vi "Motor Transfer.vi"() -> ()   [LabVIEW 2017]
panel:
  in  "Transfer Function Paramters":T1(array[cluster])=[{"Positive"={"Slope"=10.938761399489797, "Intercept"=-2.8907221360051634}, "Negative"={"Slope"=10.353560585244502, "Intercept"=2.6844501013936566}}, {"Positive"={"Slope"=10.727962252753825, "Intercept"=-2.8448867369446544}, "Negative"={"Slope"=10.977250586448044, "Intercept"=2.8878306079303058}}]
  # "Left Wheel"
  # "Right Wheel"
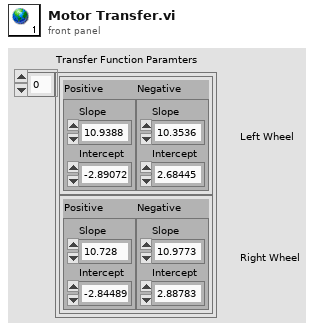
[diagram p1: front panel]
types:
  T1 = cluster{"Positive":cluster{"Slope":dbl, "Intercept":dbl}, "Negative":cluster{"Slope":dbl, "Intercept":dbl}}[]
diagram:
